vi "Add.vi"(4 "Self":variant, 6 "Parent ID (0)":i32, 8 "error in (no error)":errorcluster, 9 "Config Section":string, 10 "Config Path":path, 11 "Name":string) -> (0 "error out":errorcluster, 3 "Module":T1)   [LabVIEW 2018, in "Core.lvlib" / "Module.lvlib"]
uses:
  Module.lvlib
  Controls/Instance.ctl
  Controls/Module.ctl
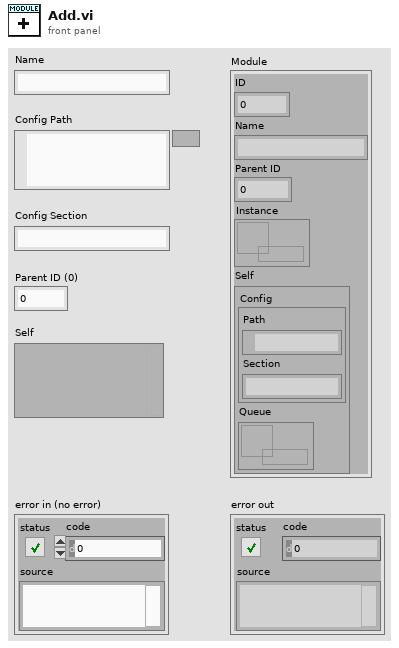
[diagram p1: front panel]
types:
  T1 = typedef "Core.lvlib/Module.lvlib/Module.ctl" = cluster{"ID":i32, "Name":string, "Parent ID":i32, "Instance":refnum<data-value>, "Self":T2}
  T2 = typedef "Core.lvlib/Module.lvlib/Instance.ctl" = cluster{"Config":cluster{"Path":path, "Section":string}, "Queue":refnum<queue>}
  T3 = cluster{"ID":i32, "Name":string, "Parent ID":i32, "Instance":refnum<data-value>}
  T4 = cluster{"ID":i32, "Name":string, "Parent ID":i32, "Instance":refnum<data-value>}[]
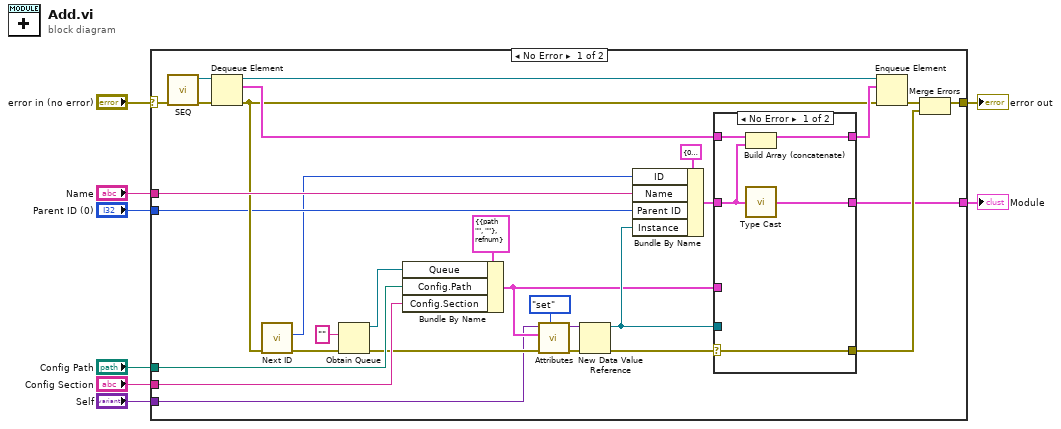
[diagram p0: block diagram]
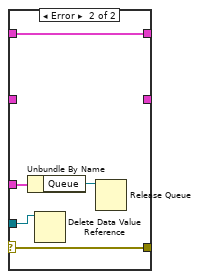
[diagram p2: hidden frame]
diagram:
  n1 = case shown="No Error" "error in (no error)" {
    selector: "error in (no error)" -> [w38 w49]
    tunnel: [w27 w49] -> w7
    tunnel: "Parent ID (0)" -> [w22 _]
    tunnel: "Name" -> [w31 _]
    tunnel: "Config Path" -> [w30 _]
    tunnel: "Config Section" -> [w29 _]
    tunnel: [w23 _] -> w2
    tunnel: "Self" -> [w10 _]
    frame No Error {
      n2 = call "SEQ.vi"("error in (no error)"=w38) -> ("error out"=w37:errorcluster, "Modules"=w36:refnum<queue>)  [unwired: 8 in, 1 out]
      n3 = Dequeue Element(queue=w36, error in (no error)=w37) -> (queue out=w34:refnum<queue>, element=w33:T4, error out=w26:errorcluster)  [unwired: 1 in, 1 out]
      n4 = call "Next ID.vi"("error in (no error)"=w26) -> ("error out"=w17:errorcluster, "Next ID"=w21:i32)  [unwired: 8 in, 1 out]
      n5 = Obtain Queue(element data type="", error in (no error)=w17) -> (queue out=w20:refnum<queue>, error out=w13:errorcluster)  [unwired: 3 in, 1 out]
      n6 = Bundle By Name(cluster=T2 {"Config"={"Path"=path "", "Section"=""}, "Queue"=refnum} ("Module Data"), "Queue"=w20, "Config.Path"=w30, "Config.Section"=w29) -> (w14:T2)
      n7 = call "Attributes.vi"("Action"=enum8{"get", "set"}."set", "error in (no error)"=w13, "Self in"=w14, "Instance in"=w10) -> ("error out"=w12:errorcluster, "Instance out"=w11:variant)  [unwired: 5 in, 1 out]
      n8 = New Data Value Reference(data value=w11, error in=w12) -> (data value reference=w15:refnum<data-value>, error out=w25:errorcluster)
      n9 = Bundle By Name(cluster=T3 {"ID"=0, "Name"="", "Parent ID"=0, "Instance"=refnum} ("Module"), "ID"=w21, "Name"=w31, "Parent ID"=w22, "Instance"=w15) -> (w28:T3)
      n10 = case shown="No Error" w25 {
        selector: w25 -> [w39 w47]
        tunnel: w33 -> [w43 w48]
        tunnel: [w42 w48] -> w32
        tunnel: w28 -> [w41 _]
        tunnel: [w39 w47] -> w24
        tunnel: [w40 _] -> w23
        tunnel: w14 -> [_ w45]
        tunnel: w15 -> [_ w44]
        frame No Error {
          n11 = Build Array (concatenate)(w43, w41) -> (w42:T4)
          n12 = call "Type Cast.vi"("Module in"=w41) -> ("Module"=w40:T1)
        }
        frame Error {
          n13 = Unbundle By Name(w45) -> ("Queue"=w46:refnum<queue>)
          n14 = Delete Data Value Reference(data value reference=w44) -> ()  [unwired: 1 in, 2 out]
          n15 = Release Queue(queue=w46) -> ()  [unwired: 2 in, 3 out]
        }
      }
      n16 = Enqueue Element(queue=w34, element=w32, error in (no error)=w26) -> (error out=w35:errorcluster)  [unwired: 1 in, 2 out]
      n17 = Merge Errors(w35, w24) -> (w27:errorcluster)
    }
    frame Error {
    }
  }
  "error out" <- w7
  "Module" <- w2
